vi "PV HLT5xx Set Pressure Data.vi"(1 "Value in":dbl=1e-09 min=1e-09 max=1000.0 step=1e-09 format="%.2e") -> (0 "Output":string)   [LabVIEW 2021, in "Pfeiffer Vacuum.lvlib"]
uses:
  <instrlib>/Pfeiffer Vacuum/Pfeiffer Vacuum.lvlib
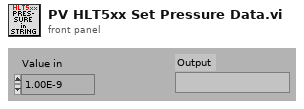
[diagram p1: front panel]
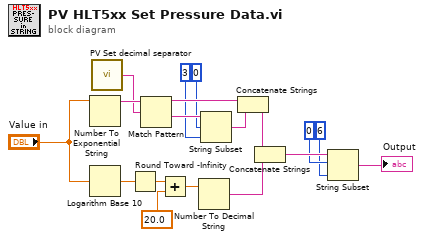
[diagram p0: block diagram]
diagram:
  n1 = Number To Exponential String(number="Value in") -> (E-format string=w13:string)  [unwired: 3 in]
  n2 = Logarithm Base 10(1:"Value in") -> (0:w16:dbl)
  n3 = call <instrlib>:"PV Set decimal separator.vi"() -> ("decimal separator"=w1:string)
  n4 = Round Toward -Infinity(1:w16) -> (0:w15:dbl)
  n5 = Match Pattern(string=w13, regular expression=w1) -> (before substring=w14:string, after substring=w12:string)  [unwired: 1 in, 2 out]
  n6 = Add(x=w15, y=20.0) -> (x+y=w8:dbl)
  n7 = Number To Decimal String(number=w8) -> (decimal integer string=w5:string)  [unwired: 1 in]
  n8 = String Subset(string=w12, offset (0)=0 ("Offset (0)"), length (rest)=3 ("Länge")) -> (substring=w9:string)
  n9 = Concatenate Strings(w14, w9) -> (w6:string)
  n10 = Concatenate Strings(w6, w5) -> (w4:string)
  n11 = String Subset(string=w4, offset (0)=0 ("Offset (0)"), length (rest)=6 ("Länge")) -> (substring=→"Output":string)
